vi "Internal Message to uService Actor Core.vi"(8 "error in (no error)":errorcluster, 9 "Message":variant, 10 "Msg Selector":T1, 11 "uService Template in":refnum<class "Father of all uServices.lvclass">) -> (0 "error out":errorcluster, 3 "uService Template out":refnum<class "Father of all uServices.lvclass">)   [LabVIEW 2026, in "TALOS.lvlib" / "Father of all uServices.lvlib" / "Father of all uServices.lvclass"]
uses:
  Father of all uServices.lvclass
  Msg to uServ Selector.ctl
  Father of all uServices.lvclass/Father of all uServices.ctl
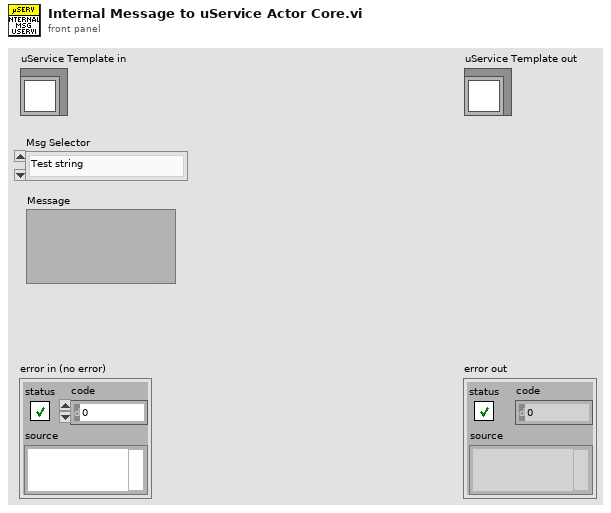
[diagram p1: front panel]
types:
  T1 = typedef "TALOS.lvlib/Father of all uServices.lvlib/Father of all uServices.lvclass/Msg to uServ Selector.ctl" = enum16{"Test string"}
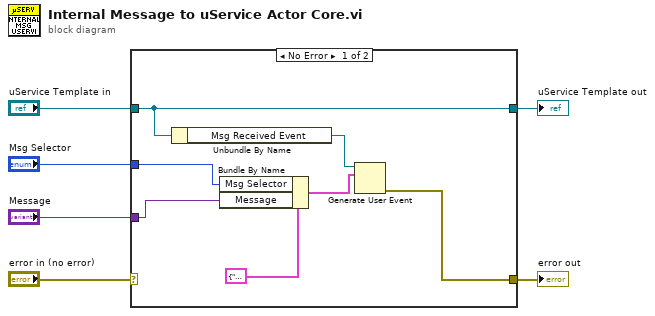
[diagram p0: block diagram]
diagram:
  n1 = case shown="No Error" "error in (no error)" {
    selector: "error in (no error)" -> [_ w15]
    tunnel: [w13 w15] -> w5
    tunnel: [w11 w14] -> w3
    tunnel: "uService Template in" -> [w11 w14]
    tunnel: "Message" -> [w8 _]
    tunnel: "Msg Selector" -> [w7 _]
    frame No Error {
      n2 = Unbundle By Name(w11) -> ("Msg Received Event"=w12:refnum<user-event>)
      n3 = Bundle By Name(cluster=cluster{"Msg Selector":T1, "Message":variant} {"Msg Selector"=enum."Test string", "Message"=variant} ("event data"), "Msg Selector"=w7, "Message"=w8) -> (w9:cluster{"Msg Selector":T1, "Message":variant})
      n4 = Generate User Event(user event=w12, event data cluster=w9) -> (error out=w13:errorcluster)  [unwired: 2 in, 1 out]
    }
    frame Error {
    }
  }
  "error out" <- w5
  "uService Template out" <- w3
